vi "Untitled 3 (SubVI).vi"(9 "Coordinates":T1, 10 "TileNumber":u16, 11 "Game in":refnum<class "Game.lvclass">) -> (3 "Game out":refnum<class "Game.lvclass">)   [LabVIEW 2019, in "RT_Game.lvlib" / "Game.lvclass"]
uses:
  Game.lvclass
  Coordinate.ctl
  Game.lvclass/Game.ctl
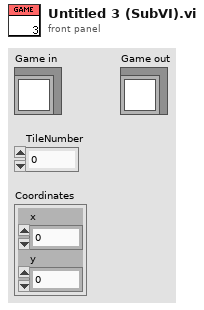
[diagram p1: front panel]
types:
  T1 = typedef "RT_Game.lvlib/Game.lvclass/Coordinate.ctl" = cluster{"x":dbl, "y":dbl}
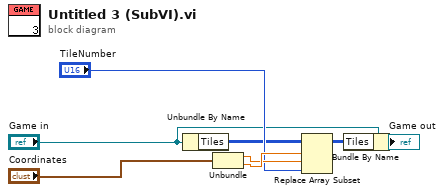
[diagram p0: block diagram]
diagram:
  n1 = Unbundle By Name("Game in") -> ("Tiles"=w2:u16[][])
  n2 = Unbundle("Coordinates") -> ("x"=w7:dbl, "y"=w8:dbl)
  n3 = Replace Array Subset(array=w2, new element="TileNumber", index (row)=w8, index (col)=w7) -> (w4:u16[][])
  n4 = Bundle By Name(cluster="Game in", "Tiles"=w4) -> (→"Game out":refnum<class "Game.lvclass">)
